vi "FiletxtOpen.vi"(6 "Tips":refnum<vi>, 7 "Language":u32, 8 "ProgressBar":refnum<vi>, 9 "ProgressNum":refnum<vi>, 10 "MessageLinCnt":refnum<vi>, 11 "file path (dialog if empty)":path caption="文件路径 （空时为对话框）") -> (0 "PathOut":path, 1 "重构的Data数组":u32[][](array[numeric]), 2 "统计数量":string[](array[string]), 3 "报文ID":string[](array[string]), 4 "BaseTimeCluster":T1, 5 "CAN报文统计":string[][](array[string]))   [LabVIEW 2015]
uses:
  <vilib>/Utility/file.llb/Read Delimited Spreadsheet (string).vi
  <vilib>/regexp/Match Regular Expression.xnode
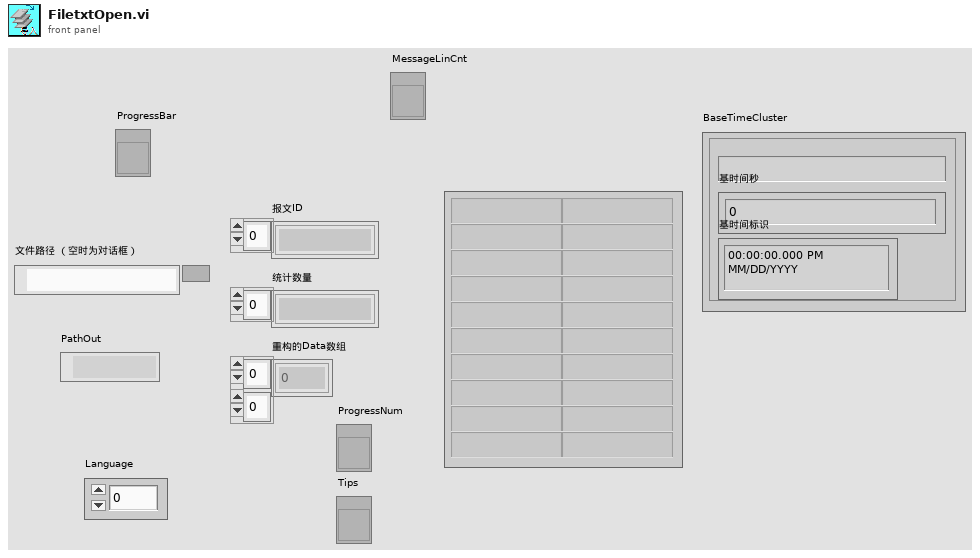
[diagram p1: front panel]
types:
  T1 = cluster{"基时间字符串":string, "基时间秒":dbl, "基时间标识":timestamp}
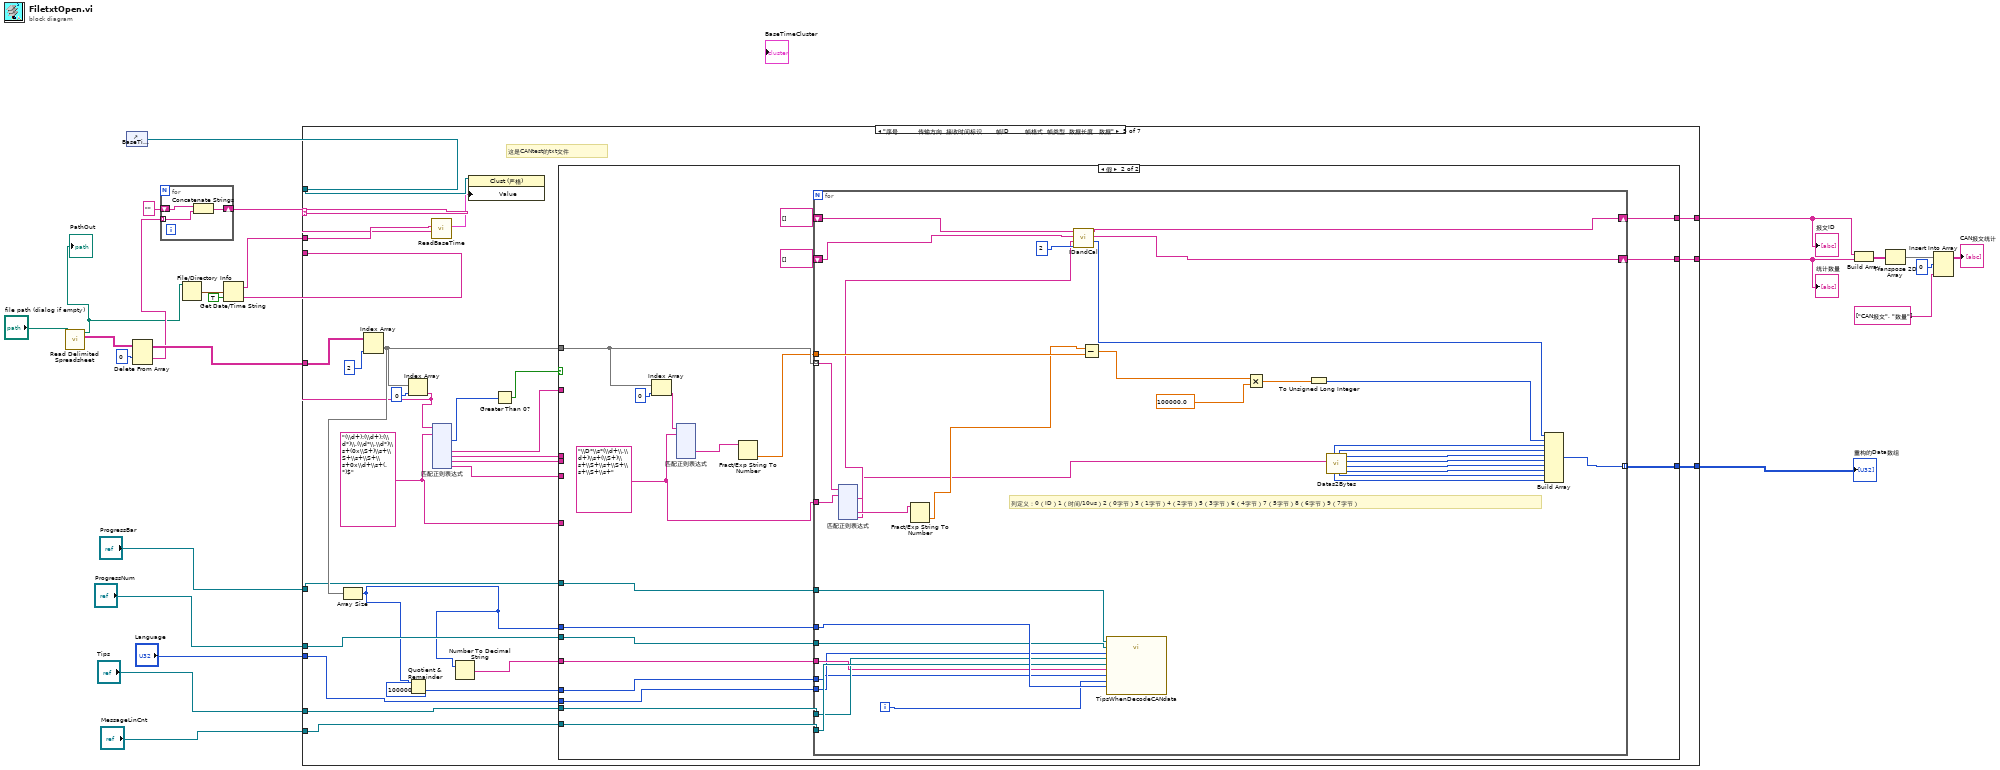
[diagram p0: block diagram]
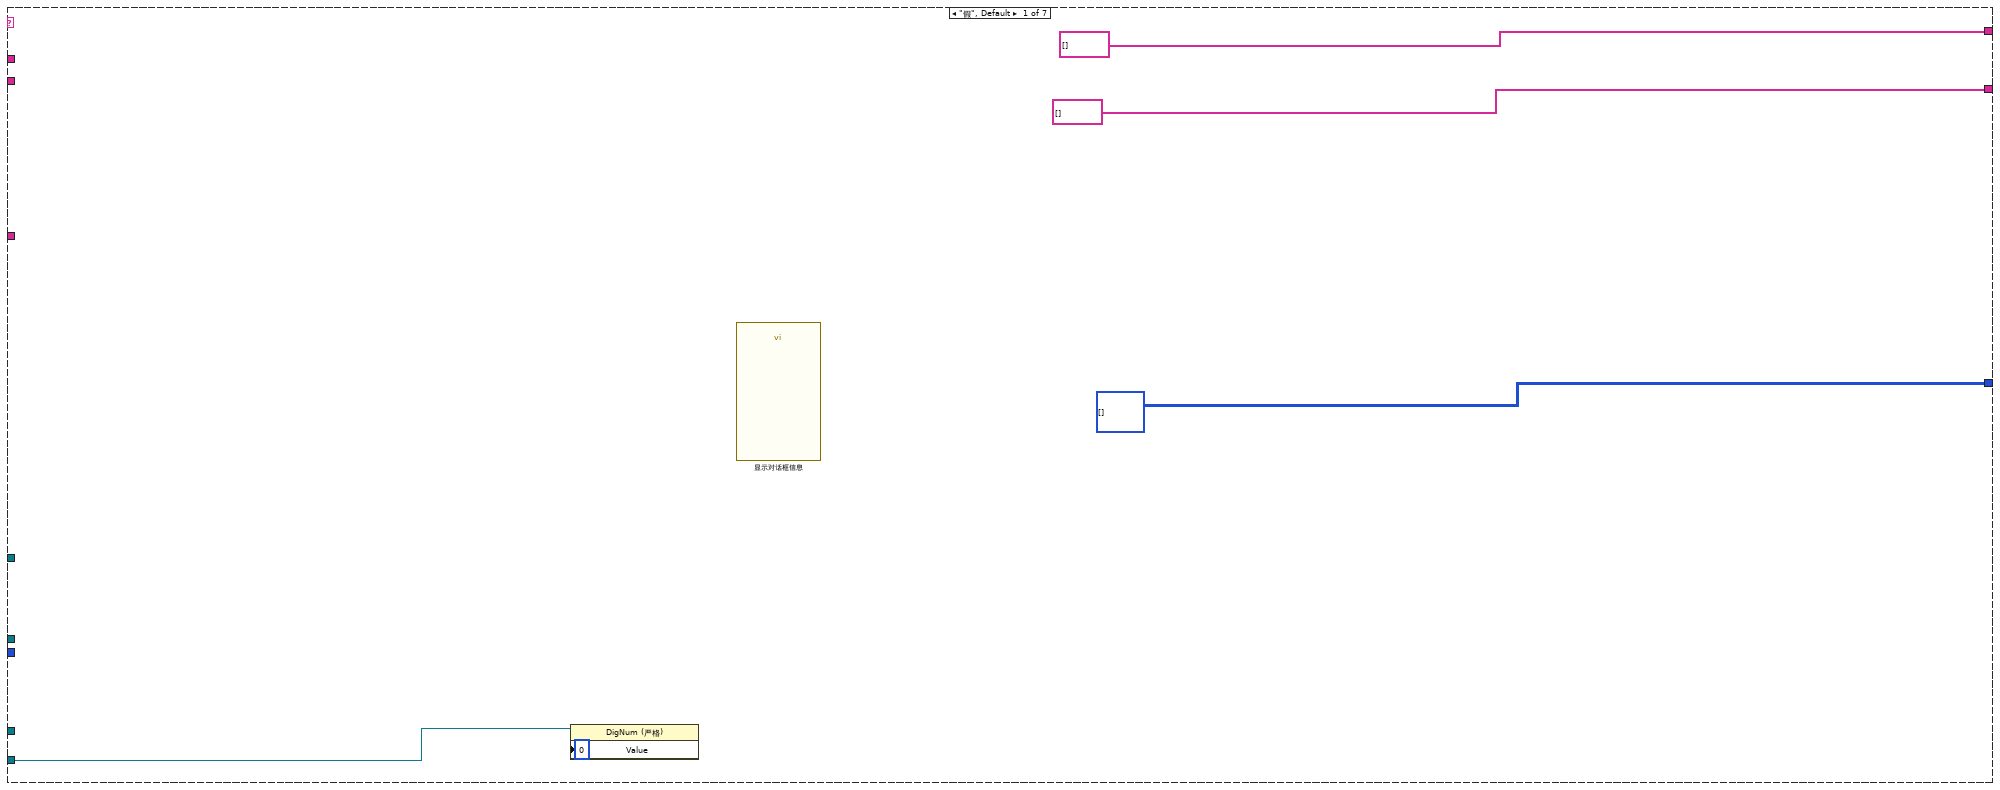
[diagram p2: hidden frame]
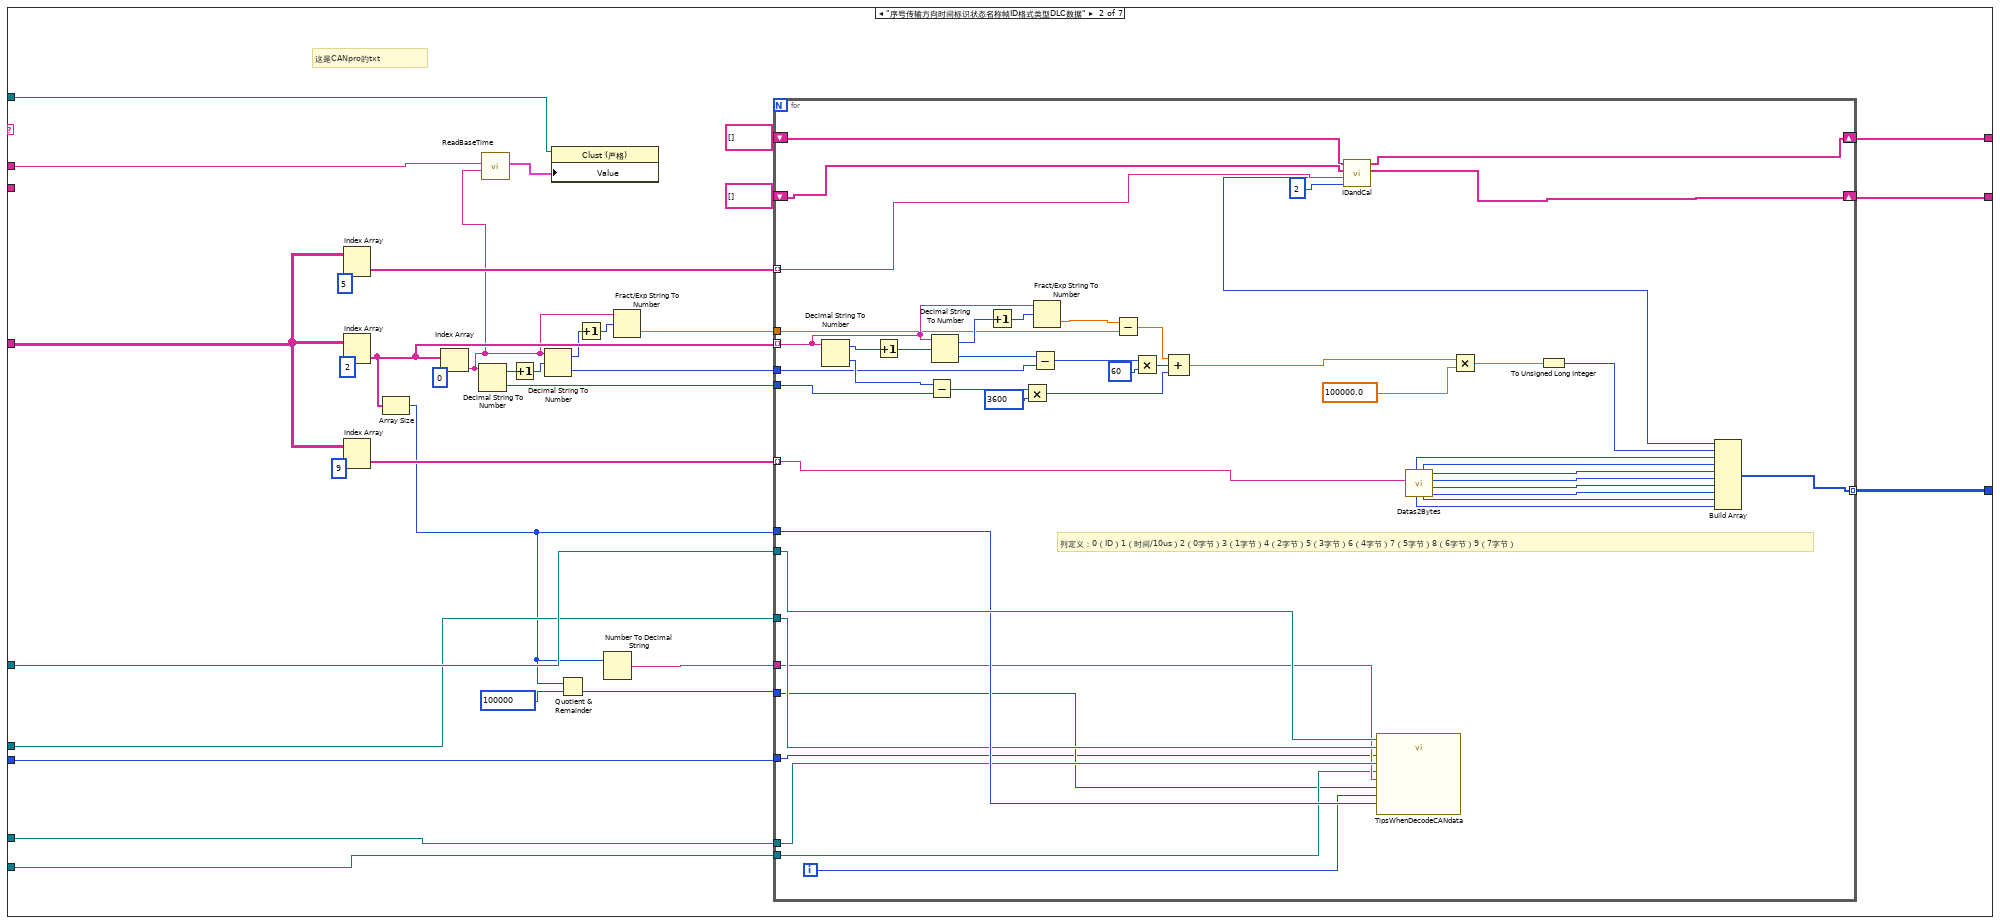
[diagram p3: hidden frame]
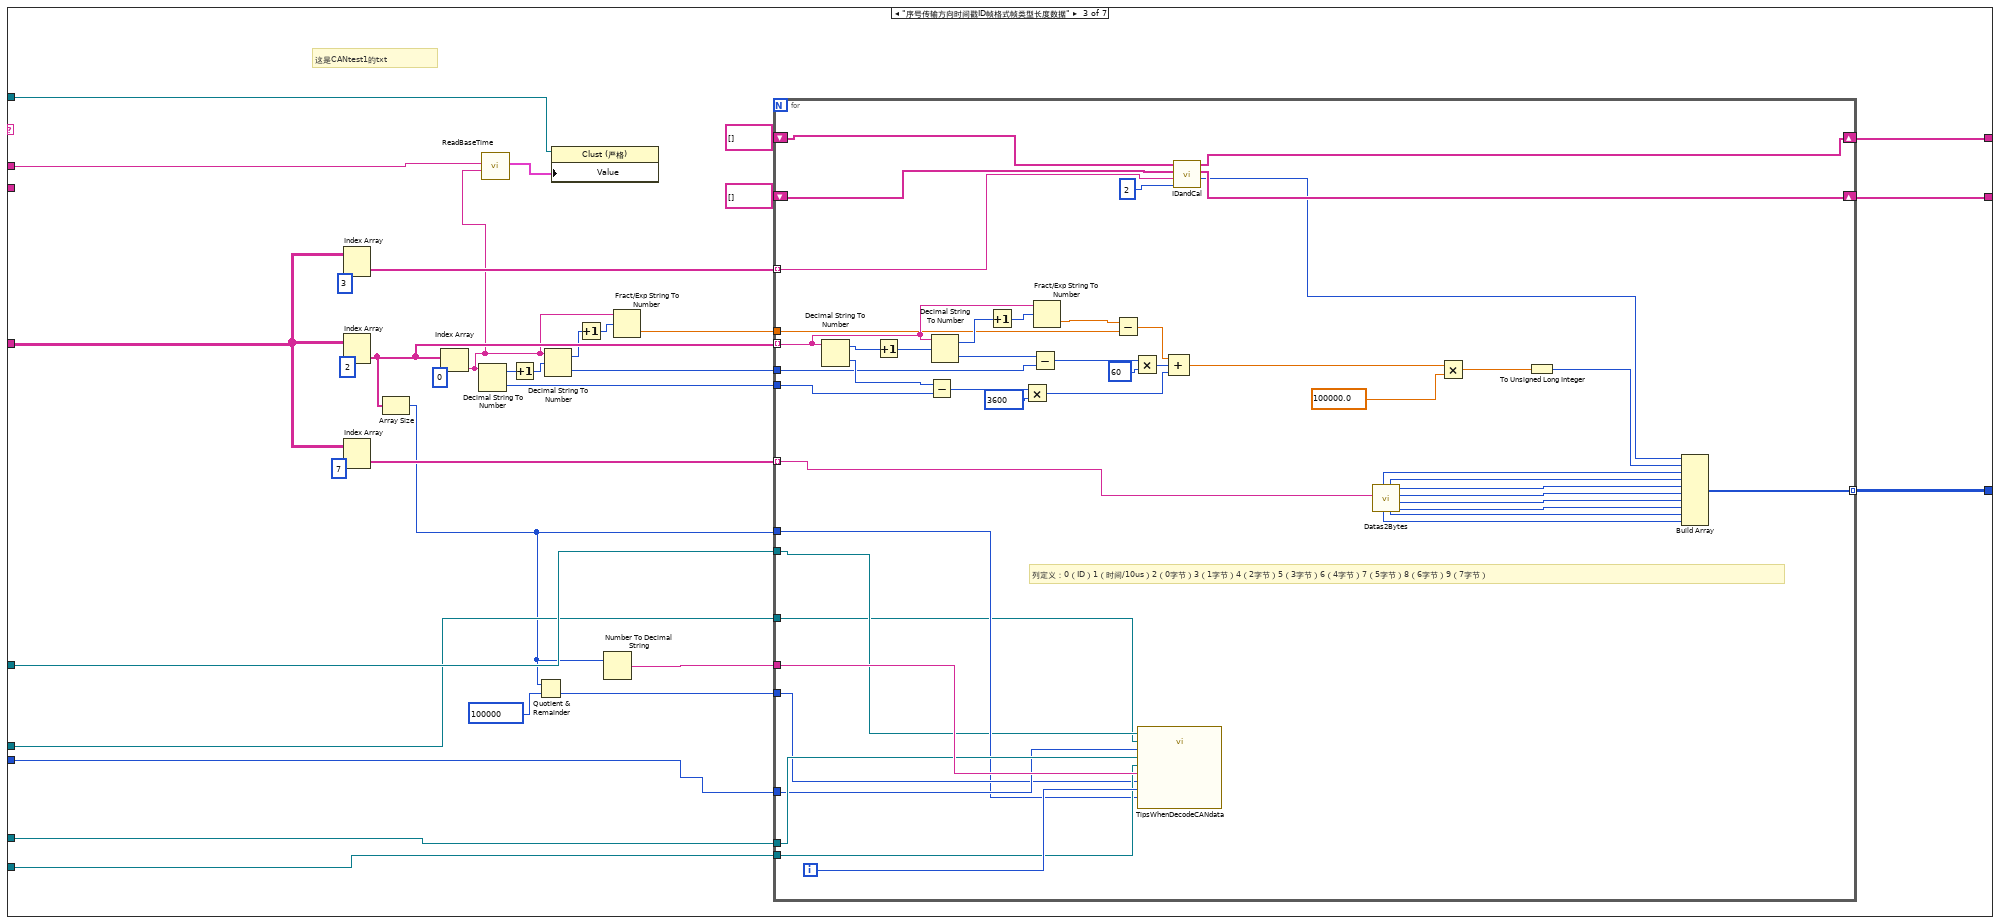
[diagram p4: hidden frame]
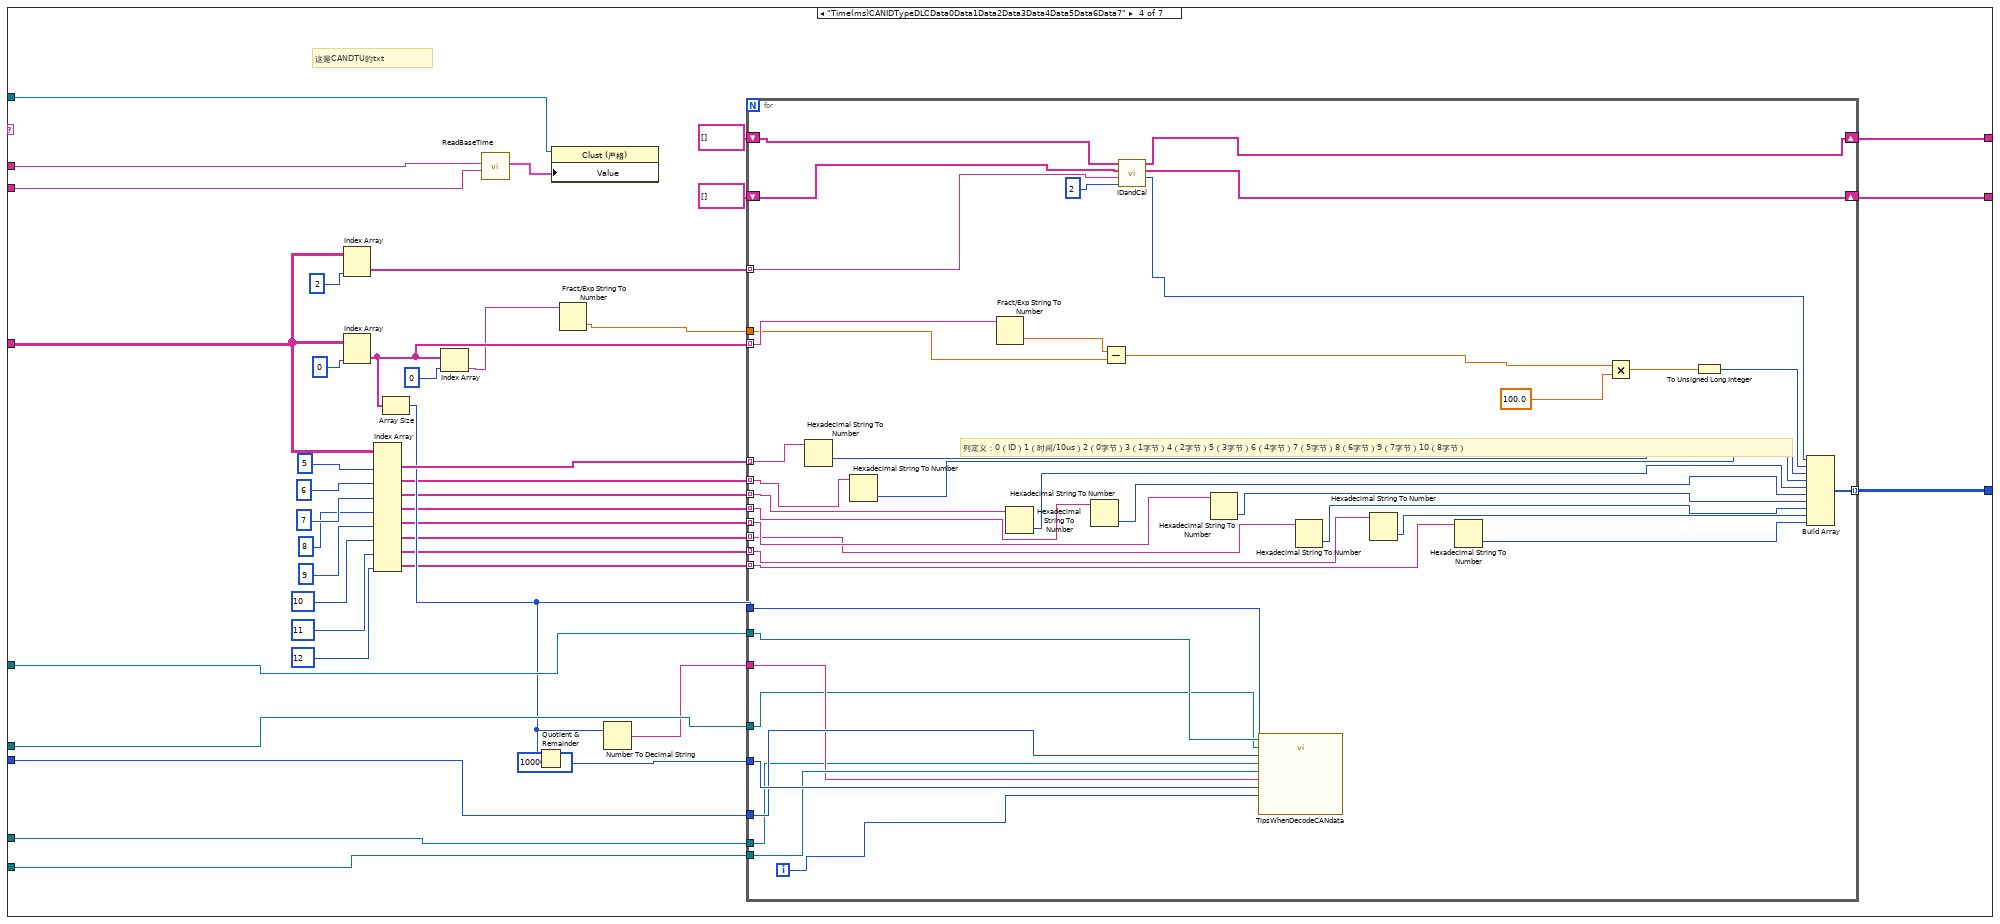
[diagram p5: hidden frame]
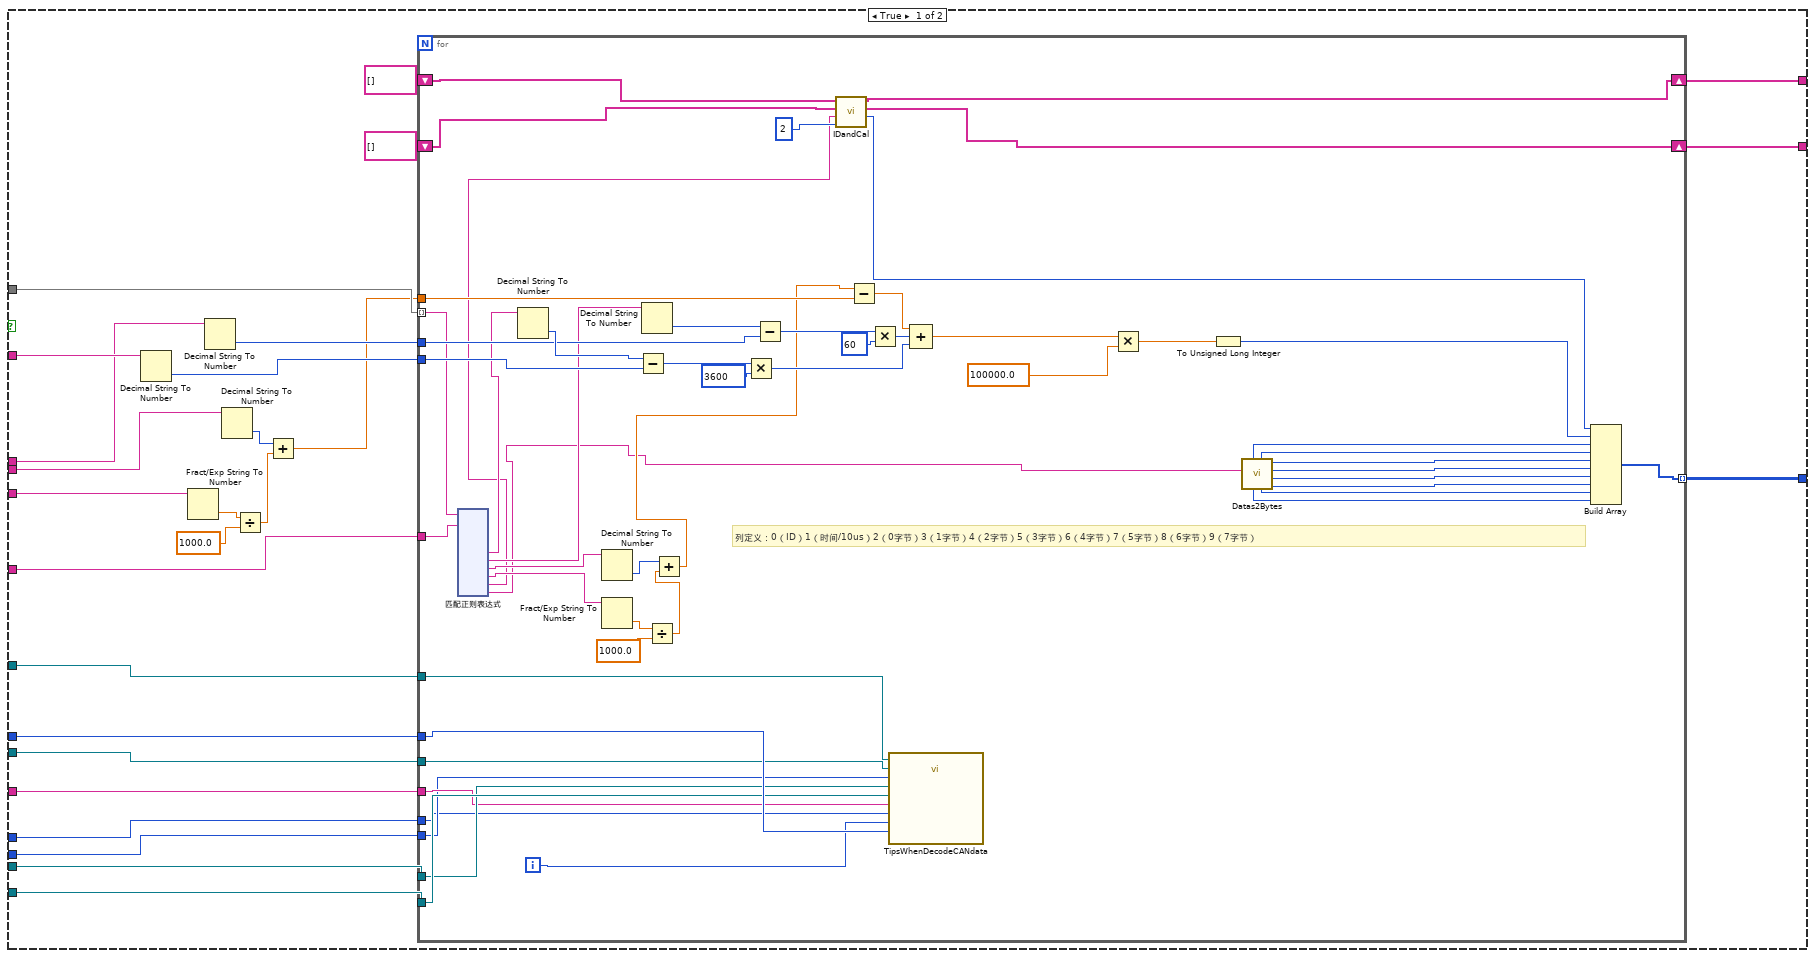
[diagram p6: hidden frame]
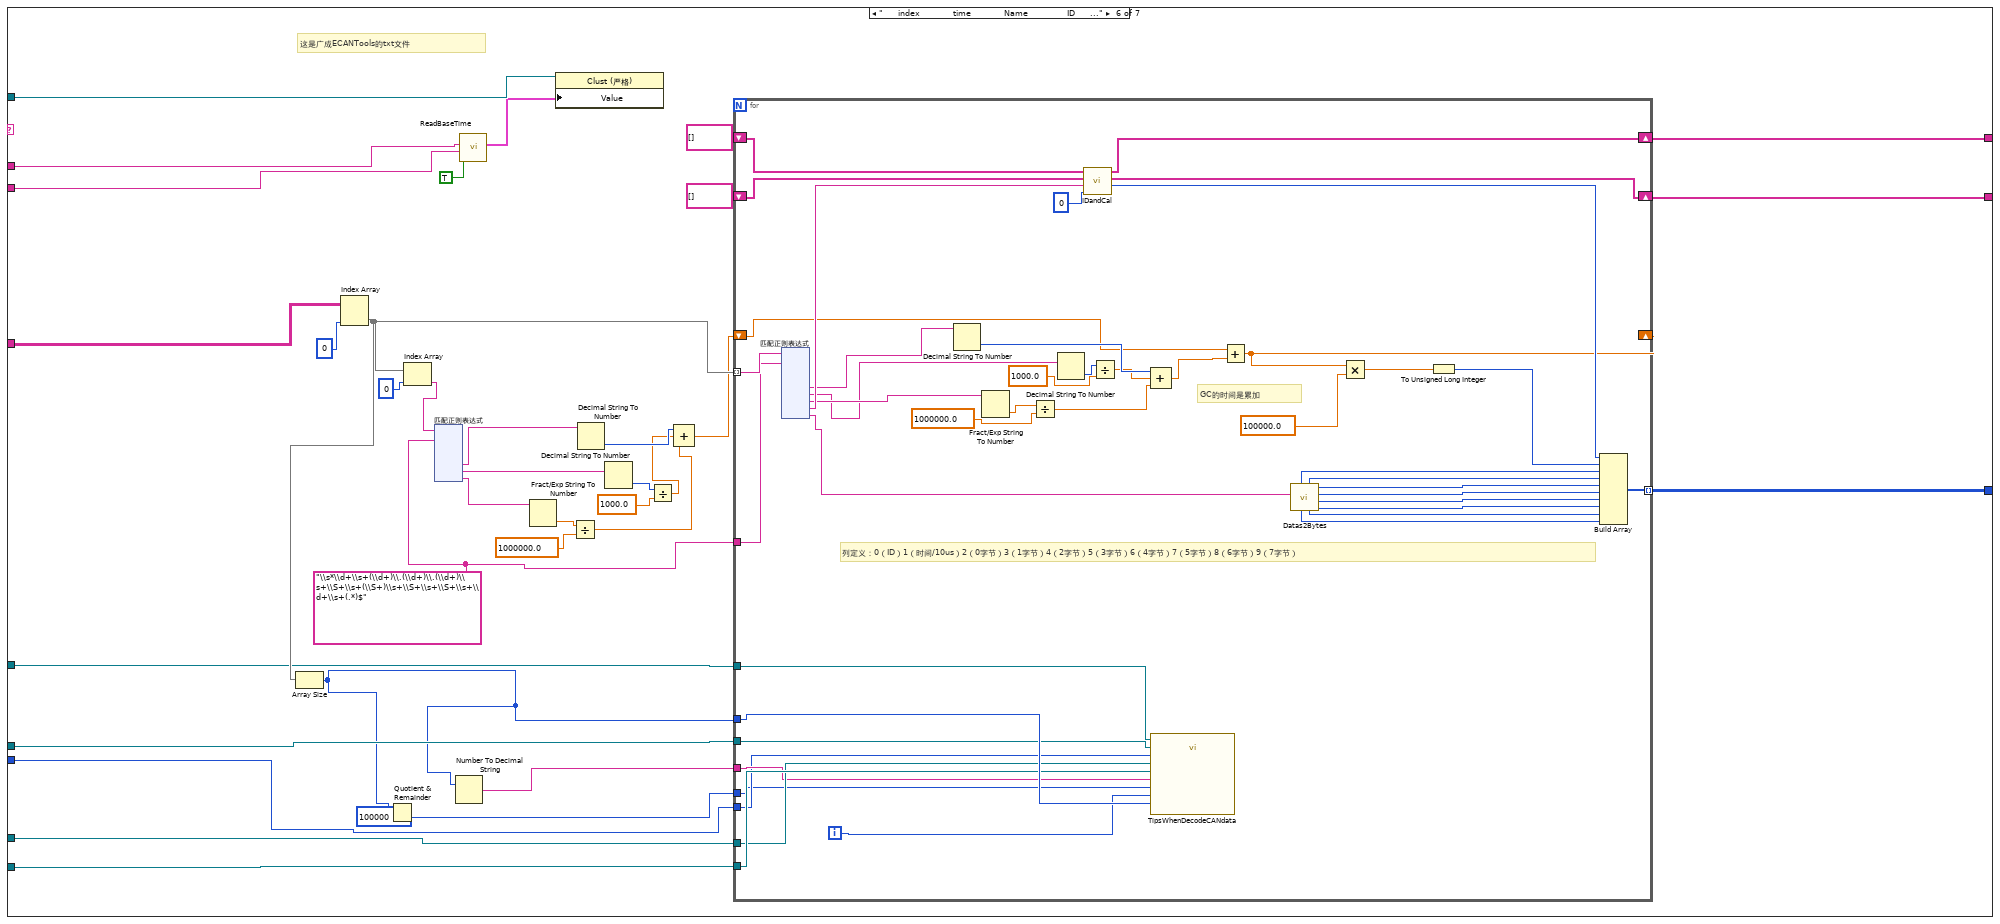
[diagram p7: hidden frame]
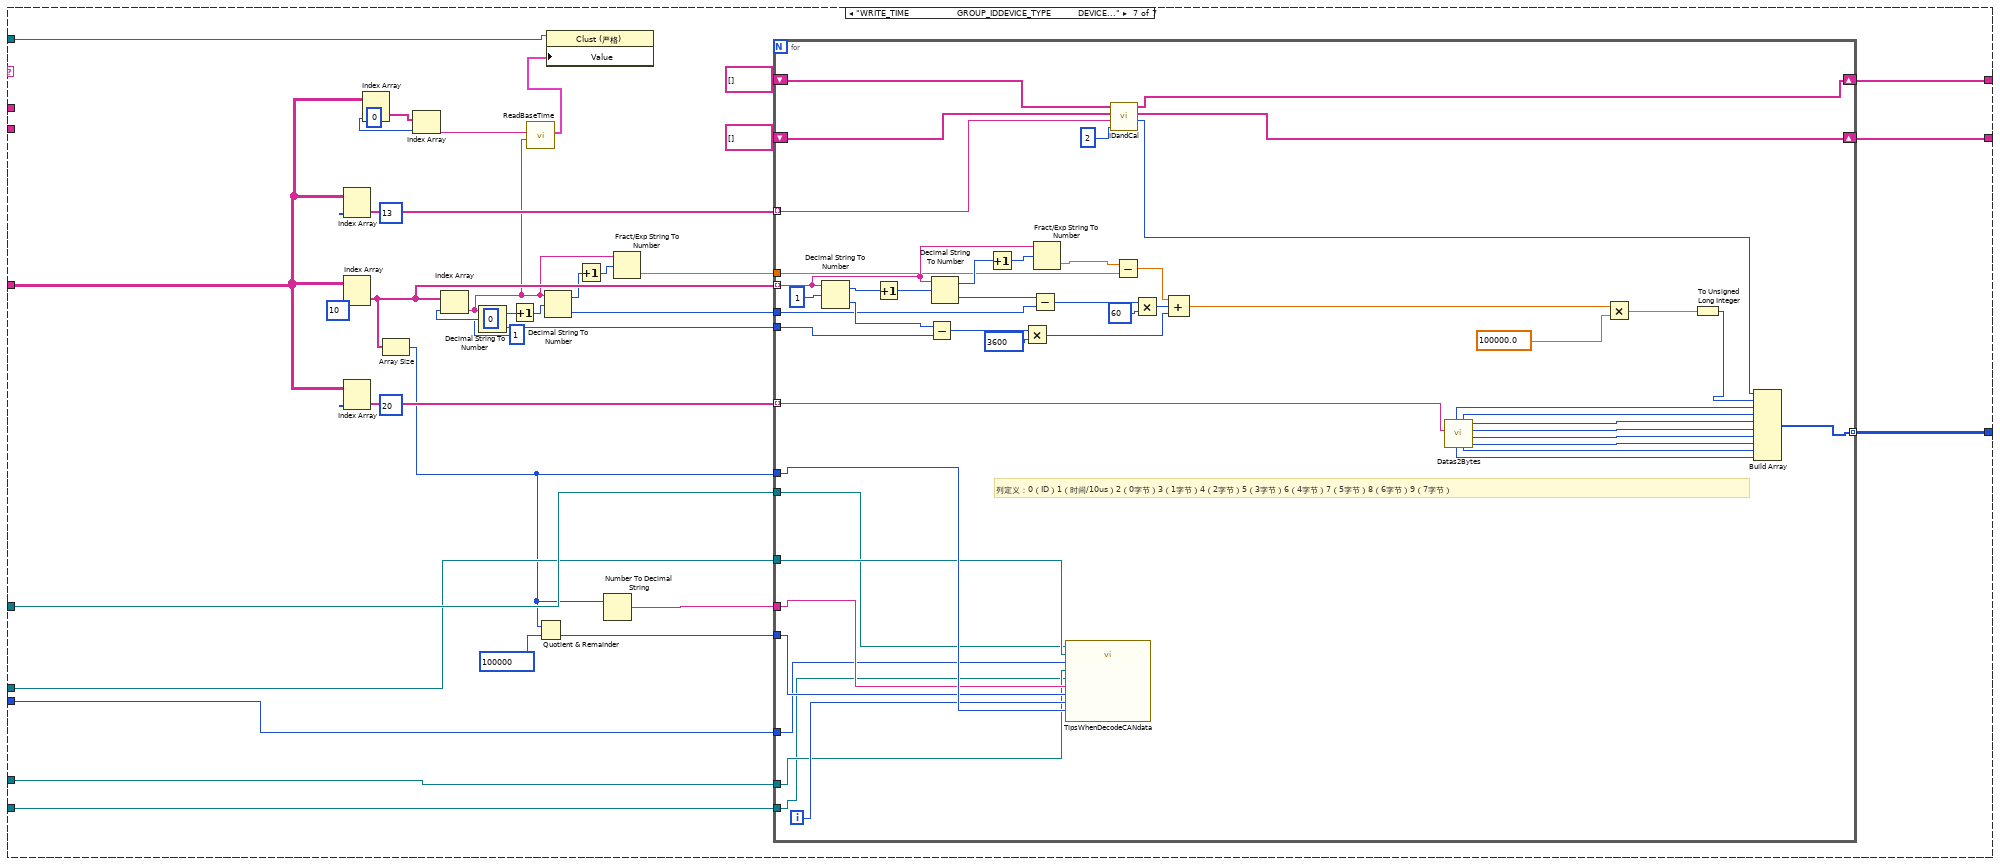
[diagram p8: hidden frame]
diagram:
  n1 = call-poly <vilib>:"Read Delimited Spreadsheet.vi"("file path (dialog if empty)"="file path (dialog if empty)") -> ("new file path (Not A Path if cancelled)"=w6:path, "all rows"=w16:string[][])  [unwired: 9 in, 4 out]
  "PathOut" <- w6
  n2 = control-ref of="BaseTimeCluster"() -> (w4:refnum<vi>)
  n3 = Delete From Array(array=w16, index (row)=0 ("索引 (行)")) -> (deleted portion=w9:string[], array with subset deleted=w25:string[][])  [unwired: 2 in]
  n4 = for {
    tunnel: w9 -> [w28] mode=indexing
    shift-right: [w29] -> w8
    shift-left: "" -> [w27]
    n5 = Concatenate Strings(w27, w28) -> (w29:string)
  }
  n6 = File/Directory Info(path=w6) -> (last mod=w7:timestamp)  [unwired: 1 in, 6 out]
  n7 = Get Date/Time String(seconds (now)=w7, want seconds? (F)=TRUE ("需要秒？(F)")) -> (date string=w5:string, time string=w3:string)  [unwired: 1 in]
  n8 = case shown="\"序号          传输方向  接收时间标识       帧ID        帧格式  帧类型  数据长度   数据\"" w8 {
    tunnel: [u32[][] [] w67 w148 w238 w305 w948 w1266] -> w26
    tunnel: w25 -> [_ w65 w146 w236 w304 w947 w1237]
    tunnel: [string[] [] w49 w130 w227 w300 w941 w1249] -> w19
    tunnel: [string[] [] w48 w129 w226 w299 w940 w1248] -> w18
    tunnel: "ProgressBar" -> [_ w47 w128 w225 w298 w939 w1247]
    tunnel: "ProgressNum" -> [_ w46 w127 w224 w297 w938 w1246]
    tunnel: "Tips" -> [_ w43 w124 w221 w294 w935 w1243]
    tunnel: "MessageLinCnt" -> [w31 w36 w117 w215 w282 w926 w1232]
    tunnel: w5 -> [_ w38 w119 w217 w286 w930 _]
    tunnel: w4 -> [_ w37 w118 w216 w284 w928 w1234]
    tunnel: w3 -> [_ _ _ w199 _ w914 _]
    tunnel: "Language" -> [_ w35 w116 w197 w281 w925 w1231]
    frame "假", Default {
      n9 = property class="DigNum (严格)"(reference=w31, "Value"=0 ("值")) -> ()  [unwired: 1 in, 2 out]
      n10 = call "显示对话框信息"() -> ()  [unwired: 10 in, 2 out]
    }
    frame "序号传输方向时间标识状态名称帧ID格式类型DLC数据" {
      # "这是CANpro的txt"
      n11 = Index Array(array=w65, index (col)=5 ("禁用的索引 (列)")) -> (element=w66:string[])  [unwired: 1 in]
      n12 = Index Array(array=w65, index (col)=2 ("禁用的索引 (列)")) -> (element=w56:string[])  [unwired: 1 in]
      n13 = Index Array(array=w65, index (col)=9 ("禁用的索引 (列)")) -> (element=w61:string[])  [unwired: 1 in]
      n14 = Array Size(array=w56) -> (size(s)=w41:i32)
      n15 = Index Array(array=w56, index=0 ("索引")) -> (element=w40:string)
      n16 = Decimal String To Number(string=w40) -> (offset past number=w53:i32, number=w57:i32)  [unwired: 2 in]
      n17 = call "ReadBaseTime.vi"("时间字符"=w40, "日期字符"=w38) -> ("基时间簇"=w39:T1)  [unwired: 7 in]
      n18 = Increment(x=w53) -> (x+1=w54:i32)
      n19 = Decimal String To Number(string=w40, offset=w54) -> (offset past number=w55:i32, number=w58:i32)  [unwired: 1 in]
      n20 = property class="Clust (严格)"(reference=w37, "Value"=w39) -> ()  [unwired: 1 in, 2 out]
      n21 = Quotient & Remainder(x=w41, y=100000) -> (floor(x/y)=w44:i32)  [unwired: 1 out]
      n22 = Increment(x=w55) -> (x+1=w59:i32)
      n23 = Number To Decimal String(number=w41) -> (decimal integer string=w42:string)  [unwired: 1 in]
      n24 = Fract/Exp String To Number(string=w40, offset=w59) -> (number=w60:dbl)  [unwired: 2 in, 1 out]
      n25 = for {
        tunnel: w56 -> [w101] mode=indexing
        tunnel: w57 -> [w111]
        tunnel: w58 -> [w107]
        tunnel: w60 -> [w99]
        tunnel: w61 -> [w68] mode=indexing
        tunnel: [w71] -> w67 mode=indexing
        shift-right: [w84] -> w49
        shift-left: string[] [] -> [w80]
        shift-right: [w85] -> w48
        shift-left: string[] [] -> [w81]
        tunnel: w66 -> [w82] mode=indexing
        tunnel: w41 -> [w93]
        tunnel: w47 -> [w94]
        tunnel: w46 -> [w92]
        tunnel: w44 -> [w87]
        tunnel: w43 -> [w91]
        tunnel: w42 -> [w90]
        tunnel: w36 -> [w89]
        tunnel: w35 -> [w86]
        i -> [w88]
        # "列定义：0（ID）1（时间/10us）2（0字节）3（1字节）4（2字节）5（3字节）6（4字节）7（5字节）8（6字节）9（7字节）"
        n26 = Decimal String To Number(string=w101) -> (offset past number=w113:i32, number=w112:i32)  [unwired: 2 in]
        n27 = Increment(x=w113) -> (x+1=w114:i32)
        n28 = Subtract(x=w112, y=w111) -> (x-y=w110:i32)
        n29 = Decimal String To Number(string=w101, offset=w114) -> (offset past number=w115:i32, number=w108:i32)  [unwired: 1 in]
        n30 = Increment(x=w115) -> (x+1=w102:i32)
        n31 = Multiply(x=w110, y=3600) -> (x*y=w103:i32)
        n32 = Subtract(x=w108, y=w107) -> (x-y=w106:i32)
        n33 = Fract/Exp String To Number(string=w101, offset=w102) -> (number=w100:dbl)  [unwired: 2 in, 1 out]
        n34 = Subtract(x=w100, y=w99) -> (x-y=w98:dbl)
        n35 = Multiply(x=w106, y=60) -> (x*y=w104:i32)
        n36 = Compound Arithmetic op=ADD(w98, w104, w103) -> (w97:dbl)
        n37 = call "IDandCal.vi"("ID列表In"=w80, "数量统计in"=w81, "ID输入"=w82, "偏移量(0)"=2) -> ("ID列表"=w84:string[], "数量统计"=w85:string[], "ID输出"=w70:u32)  [unwired: 3 in]
        n38 = call "TipsWhenDecodeCANdata.vi"("ProgressBar"=w94, "AllRowsNum"=w93, "i"=w88, "ProgressNum"=w92, "Language"=w86, "Tips"=w91, "MessageLinCnt"=w89, "txtAllRowsNum"=w90, "RowsLevel"=w87) -> ()  [unwired: 7 in]
        n39 = call "Datas2Bytes.vi"("DATAs"=w68) -> ("Data5"=w74:u32, "Data4"=w75:u32, "Data3"=w76:u32, "Data2"=w77:u32, "Data6"=w73:u32, "Data1"=w78:u32, "Data7"=w72:u32, "Data0"=w79:u32)  [unwired: 3 in]
        n40 = Multiply(x=w97, y=100000.0) -> (x*y=w95:dbl)
        n41 = To Unsigned Long Integer(number=w95) -> (unsigned 32bit integer=w69:u32)
        n42 = Build Array(w70, w69, w79, w78, w77, w76, w75, w74, w73, w72) -> (w71:u32[])
      }
    }
    frame "序号传输方向时间戳ID帧格式帧类型长度数据" {
      # "这是CANtest1的txt"
      n43 = Index Array(array=w146, index (col)=3 ("禁用的索引 (列)")) -> (element=w147:string[])  [unwired: 1 in]
      n44 = Index Array(array=w146, index (col)=2 ("禁用的索引 (列)")) -> (element=w137:string[])  [unwired: 1 in]
      n45 = Index Array(array=w146, index (col)=7 ("禁用的索引 (列)")) -> (element=w142:string[])  [unwired: 1 in]
      n46 = Array Size(array=w137) -> (size(s)=w122:i32)
      n47 = Index Array(array=w137, index=0 ("索引")) -> (element=w121:string)
      n48 = Decimal String To Number(string=w121) -> (offset past number=w134:i32, number=w138:i32)  [unwired: 2 in]
      n49 = call "ReadBaseTime.vi"("时间字符"=w121, "日期字符"=w119) -> ("基时间簇"=w120:T1)  [unwired: 7 in]
      n50 = Increment(x=w134) -> (x+1=w135:i32)
      n51 = Quotient & Remainder(x=w122, y=100000) -> (floor(x/y)=w125:i32)  [unwired: 1 out]
      n52 = Decimal String To Number(string=w121, offset=w135) -> (offset past number=w136:i32, number=w139:i32)  [unwired: 1 in]
      n53 = property class="Clust (严格)"(reference=w118, "Value"=w120) -> ()  [unwired: 1 in, 2 out]
      n54 = Increment(x=w136) -> (x+1=w140:i32)
      n55 = Number To Decimal String(number=w122) -> (decimal integer string=w123:string)  [unwired: 1 in]
      n56 = Fract/Exp String To Number(string=w121, offset=w140) -> (number=w141:dbl)  [unwired: 2 in, 1 out]
      n57 = for {
        tunnel: w137 -> [w182] mode=indexing
        tunnel: w138 -> [w192]
        tunnel: w139 -> [w188]
        tunnel: w141 -> [w180]
        tunnel: w142 -> [w149] mode=indexing
        tunnel: [w152] -> w148 mode=indexing
        shift-right: [w164] -> w130
        shift-left: string[] [] -> [w162]
        shift-right: [w163] -> w129
        shift-left: string[] [] -> [w161]
        tunnel: w147 -> [w165] mode=indexing
        tunnel: w122 -> [w169]
        tunnel: w128 -> [w168]
        tunnel: w127 -> [w167]
        tunnel: w125 -> [w170]
        tunnel: w124 -> [w172]
        tunnel: w123 -> [w175]
        tunnel: w117 -> [w173]
        tunnel: w116 -> [w171]
        i -> [w174]
        # "列定义：0（ID）1（时间/10us）2（0字节）3（1字节）4（2字节）5（3字节）6（4字节）7（5字节）8（6字节）9（7字节）"
        n58 = Decimal String To Number(string=w182) -> (offset past number=w194:i32, number=w193:i32)  [unwired: 2 in]
        n59 = Increment(x=w194) -> (x+1=w195:i32)
        n60 = Subtract(x=w193, y=w192) -> (x-y=w191:i32)
        n61 = Decimal String To Number(string=w182, offset=w195) -> (offset past number=w196:i32, number=w189:i32)  [unwired: 1 in]
        n62 = Increment(x=w196) -> (x+1=w183:i32)
        n63 = Multiply(x=w191, y=3600) -> (x*y=w184:i32)
        n64 = Subtract(x=w189, y=w188) -> (x-y=w187:i32)
        n65 = Fract/Exp String To Number(string=w182, offset=w183) -> (number=w181:dbl)  [unwired: 2 in, 1 out]
        n66 = Subtract(x=w181, y=w180) -> (x-y=w179:dbl)
        n67 = Multiply(x=w187, y=60) -> (x*y=w185:i32)
        n68 = call "TipsWhenDecodeCANdata.vi"("ProgressBar"=w168, "AllRowsNum"=w169, "i"=w174, "ProgressNum"=w167, "Language"=w171, "Tips"=w172, "MessageLinCnt"=w173, "txtAllRowsNum"=w175, "RowsLevel"=w170) -> ()  [unwired: 7 in]
        n69 = Compound Arithmetic op=ADD(w179, w185, w184) -> (w178:dbl)
        n70 = call "IDandCal.vi"("ID列表In"=w162, "数量统计in"=w161, "ID输入"=w165, "偏移量(0)"=2) -> ("ID列表"=w164:string[], "数量统计"=w163:string[], "ID输出"=w151:u32)  [unwired: 3 in]
        n71 = call "Datas2Bytes.vi"("DATAs"=w149) -> ("Data5"=w155:u32, "Data4"=w156:u32, "Data3"=w157:u32, "Data2"=w158:u32, "Data6"=w154:u32, "Data1"=w159:u32, "Data7"=w153:u32, "Data0"=w160:u32)  [unwired: 3 in]
        n72 = Multiply(x=w178, y=100000.0) -> (x*y=w176:dbl)
        n73 = To Unsigned Long Integer(number=w176) -> (unsigned 32bit integer=w150:u32)
        n74 = Build Array(w151, w150, w160, w159, w158, w157, w156, w155, w154, w153) -> (w152:u32[])
      }
    }
    frame "Time(ms)CANIDTypeDLCData0Data1Data2Data3Data4Data5Data6Data7" {
      # "这是CANDTU的txt"
      n75 = Index Array(array=w236, index (col)=2 ("禁用的索引 (列)")) -> (element=w237:string[])  [unwired: 1 in]
      n76 = Index Array(array=w236, index (col)=0 ("禁用的索引 (列)")) -> (element=w231:string[])  [unwired: 1 in]
      n77 = Index Array(array=w236, index (col) #1=5 ("禁用的索引 (列)"), index (col) #2=6 ("禁用的索引 (列)"), index (col) #3=7 ("禁用的索引 (列)"), index (col) #4=8 ("禁用的索引 (列)"), index (col) #5=9 ("禁用的索引 (列)"), index (col) #6=10 ("禁用的索引 (列)"), index (col) #7=11 ("禁用的索引 (列)"), index (col) #8=12 ("禁用的索引 (列)")) -> (element #1=w232:string[], element #2=w207:string[], element #3=w206:string[], element #4=w205:string[], element #5=w204:string[], element #6=w203:string[], element #7=w202:string[], element #8=w201:string[])  [unwired: 8 in]
      n78 = Array Size(array=w231) -> (size(s)=w219:i32)
      n79 = Index Array(array=w231, index=0 ("索引")) -> (element=w198:string)
      n80 = call "ReadBaseTime.vi"("时间字符"=w199, "日期字符"=w217) -> ("基时间簇"=w218:T1)  [unwired: 7 in]
      n81 = Quotient & Remainder(x=w219, y=100000) -> (floor(x/y)=w222:i32)  [unwired: 1 out]
      n82 = property class="Clust (严格)"(reference=w216, "Value"=w218) -> ()  [unwired: 1 in, 2 out]
      n83 = Fract/Exp String To Number(string=w198) -> (number=w200:dbl)  [unwired: 3 in, 1 out]
      n84 = Number To Decimal String(number=w219) -> (decimal integer string=w220:string)  [unwired: 1 in]
      n85 = for {
        tunnel: w231 -> [w278] mode=indexing
        tunnel: w200 -> [w276]
        tunnel: w232 -> [w263] mode=indexing
        tunnel: [w267] -> w238 mode=indexing
        shift-right: [w243] -> w227
        shift-left: string[] [] -> [w242]
        shift-right: [w244] -> w226
        shift-left: string[] [] -> [w240]
        tunnel: w237 -> [w241] mode=indexing
        tunnel: w219 -> [w254]
        tunnel: w225 -> [w247]
        tunnel: w224 -> [w246]
        tunnel: w222 -> [w252]
        tunnel: w221 -> [w248]
        tunnel: w220 -> [w249]
        tunnel: w215 -> [w250]
        tunnel: w207 -> [w262] mode=indexing
        tunnel: w206 -> [w261] mode=indexing
        tunnel: w205 -> [w260] mode=indexing
        tunnel: w204 -> [w259] mode=indexing
        tunnel: w203 -> [w258] mode=indexing
        tunnel: w202 -> [w257] mode=indexing
        tunnel: w201 -> [w256] mode=indexing
        tunnel: w197 -> [w251]
        i -> [w253]
        # "列定义：0（ID）1（时间/10us）2（0字节）3（1字节）4（2字节）5（3字节）6（4字节）7（5字节）8（6字节）9（7字节）10（8字节）"
        n86 = Hexadecimal String To Number(string=w263) -> (number=w275:u32)  [unwired: 2 in, 1 out]
        n87 = Hexadecimal String To Number(string=w262) -> (number=w274:u32)  [unwired: 2 in, 1 out]
        n88 = Fract/Exp String To Number(string=w278) -> (number=w277:dbl)  [unwired: 3 in, 1 out]
        n89 = Hexadecimal String To Number(string=w261) -> (number=w273:u32)  [unwired: 2 in, 1 out]
        n90 = Hexadecimal String To Number(string=w260) -> (number=w272:u32)  [unwired: 2 in, 1 out]
        n91 = Subtract(x=w277, y=w276) -> (x-y=w255:dbl)
        n92 = call "IDandCal.vi"("ID列表In"=w242, "数量统计in"=w240, "ID输入"=w241, "偏移量(0)"=2) -> ("ID列表"=w243:string[], "数量统计"=w244:string[], "ID输出"=w239:u32)  [unwired: 3 in]
        n93 = Hexadecimal String To Number(string=w259) -> (number=w271:u32)  [unwired: 2 in, 1 out]
        n94 = call "TipsWhenDecodeCANdata.vi"("ProgressBar"=w247, "AllRowsNum"=w254, "i"=w253, "ProgressNum"=w246, "Language"=w251, "Tips"=w248, "MessageLinCnt"=w250, "txtAllRowsNum"=w249, "RowsLevel"=w252) -> ()  [unwired: 7 in]
        n95 = Hexadecimal String To Number(string=w258) -> (number=w270:u32)  [unwired: 2 in, 1 out]
        n96 = Hexadecimal String To Number(string=w257) -> (number=w269:u32)  [unwired: 2 in, 1 out]
        n97 = Hexadecimal String To Number(string=w256) -> (number=w268:u32)  [unwired: 2 in, 1 out]
        n98 = Multiply(x=w255, y=100.0) -> (x*y=w265:dbl)
        n99 = To Unsigned Long Integer(number=w265) -> (unsigned 32bit integer=w264:u32)
        n100 = Build Array(w239, w264, w275, w274, w273, w272, w271, w270, w269, w268) -> (w267:u32[])
      }
    }
    frame "序号          传输方向  接收时间标识       帧ID        帧格式  帧类型  数据长度   数据" {
      w287 = "(\\d+):(\\d+):(\\d*)\\.(\\d*\\.\\d*)\\s+(0x\\S+)\\s+\\S+\\s+\\S+\\s+0x\\d+\\s+(.*)$"
      # "这是CANtest的txt文件"
      n101 = Index Array(array=w304, index (col)=2 ("禁用的索引 (列)")) -> (element=w303:string[])  [unwired: 1 in]
      n102 = Array Size(array=w303) -> (size(s)=w292:i32)
      n103 = Index Array(array=w303, index=0 ("索引")) -> (element=w285:string)
      n104 = Quotient & Remainder(x=w292, y=100000) -> (floor(x/y)=w295:i32)  [unwired: 1 out]
      n105 = call "ReadBaseTime.vi"("时间字符"=w285, "日期字符"=w286) -> ("基时间簇"=w283:T1)  [unwired: 7 in]
      n106 = xnode "匹配正则表达式"("输入字符串"=w285, "正则表达式"=w287) -> ("匹配后偏移量"=w280:i32, "子匹配 1"=w291:string, "子匹配 2"=w290:string, "子匹配 3"=w289:string, "子匹配 4"=w288:string)  [unwired: 4 in, 4 out]
      n107 = Number To Decimal String(number=w292) -> (decimal integer string=w293:string)  [unwired: 1 in]
      n108 = property class="Clust (严格)"(reference=w284, "Value"=w283) -> ()  [unwired: 1 in, 2 out]
      n109 = Greater Than 0?(x=w280) -> (x > 0?=w279:bool)
      n110 = case shown="假" w279 {
        tunnel: [w331 w524] -> w305
        tunnel: w303 -> [w326 w509]
        tunnel: [w325 w521] -> w300
        tunnel: [w324 w520] -> w299
        tunnel: w298 -> [w323 w519]
        tunnel: w297 -> [w322 w518]
        tunnel: w295 -> [w321 w517]
        tunnel: w294 -> [w320 w516]
        tunnel: w293 -> [w319 w515]
        tunnel: w292 -> [w318 w514]
        tunnel: w291 -> [w317 _]
        tunnel: w290 -> [w316 _]
        tunnel: w289 -> [w315 _]
        tunnel: w288 -> [w314 _]
        tunnel: w287 -> [w308 _]
        tunnel: w282 -> [w307 w513]
        tunnel: w281 -> [w306 w512]
        frame True {
          n111 = Decimal String To Number(string=w317) -> (number=w327:i32)  [unwired: 2 in, 1 out]
          n112 = Fract/Exp String To Number(string=w314) -> (number=w312:dbl)  [unwired: 3 in, 1 out]
          n113 = Decimal String To Number(string=w316) -> (number=w328:i32)  [unwired: 2 in, 1 out]
          n114 = Decimal String To Number(string=w315) -> (number=w309:i32)  [unwired: 2 in, 1 out]
          n115 = Divide(x=w312, y=1000.0) -> (x/y=w310:dbl)
          n116 = Add(x=w309, y=w310) -> (x+y=w313:dbl)
          n117 = for {
            tunnel: w326 -> [w369] mode=indexing
            tunnel: w327 -> [w383]
            tunnel: w328 -> [w379]
            tunnel: w313 -> [w374]
            tunnel: [w335] -> w331 mode=indexing
            shift-right: [w347] -> w325
            shift-left: string[] [] -> [w346]
            shift-right: [w348] -> w324
            shift-left: string[] [] -> [w345]
            tunnel: w318 -> [w358]
            tunnel: w323 -> [w350]
            tunnel: w322 -> [w351]
            tunnel: w321 -> [w352]
            tunnel: w320 -> [w355]
            tunnel: w319 -> [w354]
            tunnel: w308 -> [w368]
            tunnel: w307 -> [w356]
            tunnel: w306 -> [w353]
            i -> [w357]
            # "列定义：0（ID）1（时间/10us）2（0字节）3（1字节）4（2字节）5（3字节）6（4字节）7（5字节）8（6字节）9（7字节）"
            n118 = xnode "匹配正则表达式"("输入字符串"=w369, "正则表达式"=w368) -> ("子匹配 1"=w367:string, "子匹配 2"=w366:string, "子匹配 3"=w365:string, "子匹配 4"=w363:string, "子匹配 5"=w344:string, "子匹配 6"=w332:string)  [unwired: 4 in, 5 out]
            n119 = Decimal String To Number(string=w367) -> (number=w384:i32)  [unwired: 2 in, 1 out]
            n120 = Decimal String To Number(string=w365) -> (number=w364:i32)  [unwired: 2 in, 1 out]
            n121 = Fract/Exp String To Number(string=w363) -> (number=w361:dbl)  [unwired: 3 in, 1 out]
            n122 = Subtract(x=w384, y=w383) -> (x-y=w382:i32)
            n123 = Decimal String To Number(string=w366) -> (number=w380:i32)  [unwired: 2 in, 1 out]
            n124 = Divide(x=w361, y=1000.0) -> (x/y=w360:dbl)
            n125 = Add(x=w364, y=w360) -> (x+y=w359:dbl)
            n126 = Multiply(x=w382, y=3600) -> (x*y=w375:i32)
            n127 = Subtract(x=w380, y=w379) -> (x-y=w378:i32)
            n128 = call "IDandCal.vi"("ID列表In"=w346, "数量统计in"=w345, "ID输入"=w344, "偏移量(0)"=2) -> ("ID列表"=w347:string[], "数量统计"=w348:string[], "ID输出"=w334:u32)  [unwired: 3 in]
            n129 = Subtract(x=w359, y=w374) -> (x-y=w373:dbl)
            n130 = Multiply(x=w378, y=60) -> (x*y=w376:i32)
            n131 = call "TipsWhenDecodeCANdata.vi"("ProgressBar"=w350, "AllRowsNum"=w358, "i"=w357, "ProgressNum"=w351, "Language"=w353, "Tips"=w355, "MessageLinCnt"=w356, "txtAllRowsNum"=w354, "RowsLevel"=w352) -> ()  [unwired: 7 in]
            n132 = Compound Arithmetic op=ADD(w373, w376, w375) -> (w372:dbl)
            n133 = Multiply(x=w372, y=100000.0) -> (x*y=w370:dbl)
            n134 = To Unsigned Long Integer(number=w370) -> (unsigned 32bit integer=w333:u32)
            n135 = call "Datas2Bytes.vi"("DATAs"=w332) -> ("Data5"=w338:u32, "Data4"=w339:u32, "Data3"=w340:u32, "Data2"=w341:u32, "Data6"=w337:u32, "Data1"=w342:u32, "Data7"=w336:u32, "Data0"=w343:u32)  [unwired: 3 in]
            n136 = Build Array(w334, w333, w343, w342, w341, w340, w339, w338, w337, w336) -> (w335:u32[])
          }
        }
        frame False {
          w508 = "\\D*\\s*(\\d+\\.\\d+)\\s+(\\S+)\\s+\\S+\\s+\\S+\\s+\\S+\\s+"
          n137 = Index Array(array=w509, index=0 ("索引")) -> (element=w511:string)
          n138 = xnode "匹配正则表达式"("输入字符串"=w511, "正则表达式"=w508) -> ("子匹配 1"=w507:string)  [unwired: 4 in, 6 out]
          n139 = Fract/Exp String To Number(string=w507) -> (number=w506:dbl)  [unwired: 3 in, 1 out]
          n140 = for {
            tunnel: w509 -> [w673] mode=indexing
            tunnel: w506 -> [w676]
            tunnel: [w649] -> w524 mode=indexing
            shift-right: [w660] -> w521
            shift-left: string[] [] -> [w659]
            shift-right: [w661] -> w520
            shift-left: string[] [] -> [w658]
            tunnel: w514 -> [w671]
            tunnel: w519 -> [w663]
            tunnel: w518 -> [w664]
            tunnel: w517 -> [w665]
            tunnel: w516 -> [w668]
            tunnel: w515 -> [w667]
            tunnel: w508 -> [w672]
            tunnel: w513 -> [w669]
            tunnel: w512 -> [w666]
            i -> [w670]
            # "列定义：0（ID）1（时间/10us）2（0字节）3（1字节）4（2字节）5（3字节）6（4字节）7（5字节）8（6字节）9（7字节）"
            n141 = xnode "匹配正则表达式"("输入字符串"=w673, "正则表达式"=w672) -> ("匹配之后"=w642:string, "子匹配 1"=w645:string, "子匹配 2"=w643:string)  [unwired: 4 in, 4 out]
            n142 = Fract/Exp String To Number(string=w645) -> (number=w644:dbl)  [unwired: 3 in, 1 out]
            n143 = call "IDandCal.vi"("ID列表In"=w659, "数量统计in"=w658, "ID输入"=w643, "偏移量(0)"=2) -> ("ID列表"=w660:string[], "数量统计"=w661:string[], "ID输出"=w648:u32)  [unwired: 3 in]
            n144 = Subtract(x=w644, y=w676) -> (x-y=w646:dbl)
            n145 = call "TipsWhenDecodeCANdata.vi"("ProgressBar"=w663, "AllRowsNum"=w671, "i"=w670, "ProgressNum"=w664, "Language"=w666, "Tips"=w668, "MessageLinCnt"=w669, "txtAllRowsNum"=w667, "RowsLevel"=w665) -> ()  [unwired: 7 in]
            n146 = Multiply(x=w646, y=100000.0) -> (x*y=w674:dbl)
            n147 = To Unsigned Long Integer(number=w674) -> (unsigned 32bit integer=w647:u32)
            n148 = call "Datas2Bytes.vi"("DATAs"=w642) -> ("Data5"=w652:u32, "Data4"=w653:u32, "Data3"=w654:u32, "Data2"=w655:u32, "Data6"=w651:u32, "Data1"=w656:u32, "Data7"=w650:u32, "Data0"=w657:u32)  [unwired: 3 in]
            n149 = Build Array(w648, w647, w657, w656, w655, w654, w653, w652, w651, w650) -> (w649:u32[])
          }
        }
      }
    }
    frame "     index           time           Name             ID        Type      Format  Len      Data" {
      w924 = "\\s*\\d+\\s+(\\d+)\\.(\\d+)\\.(\\d+)\\s+\\S+\\s+(\\S+)\\s+\\S+\\s+\\S+\\s+\\d+\\s+(.*)$"
      # "这是广成ECANTools的txt文件"
      n150 = Index Array(array=w947, index (col)=0 ("禁用的索引 (列)")) -> (element=w944:string[])  [unwired: 1 in]
      n151 = Array Size(array=w944) -> (size(s)=w933:i32)
      n152 = Quotient & Remainder(x=w933, y=100000) -> (floor(x/y)=w936:i32)  [unwired: 1 out]
      n153 = Index Array(array=w944, index=0 ("索引")) -> (element=w929:string)
      n154 = xnode "匹配正则表达式"("输入字符串"=w929, "正则表达式"=w924) -> ("子匹配 1"=w923:string, "子匹配 2"=w921:string, "子匹配 3"=w917:string)  [unwired: 4 in, 5 out]
      n155 = Number To Decimal String(number=w933) -> (decimal integer string=w934:string)  [unwired: 1 in]
      n156 = call "ReadBaseTime.vi"("文件时间？(F)"=TRUE ("文件时间？"), "时间字符"=w914, "日期字符"=w930) -> ("基时间簇"=w927:T1)  [unwired: 6 in]
      n157 = Fract/Exp String To Number(string=w917) -> (number=w932:dbl)  [unwired: 3 in, 1 out]
      n158 = property class="Clust (严格)"(reference=w928, "Value"=w927) -> ()  [unwired: 1 in, 2 out]
      n159 = Divide(x=w932, y=1000000.0) -> (x/y=w916:dbl)
      n160 = Decimal String To Number(string=w923) -> (number=w922:i32)  [unwired: 2 in, 1 out]
      n161 = Decimal String To Number(string=w921) -> (number=w919:i32)  [unwired: 2 in, 1 out]
      n162 = Divide(x=w919, y=1000.0) -> (x/y=w918:dbl)
      n163 = Compound Arithmetic op=ADD(w922, w918, w916) -> (w915:dbl)
      n164 = for {
        tunnel: w944 -> [w1100] mode=indexing
        tunnel: [w1110] -> w948 mode=indexing
        shift-right: [w1105] -> w941
        shift-left: string[] [] -> [w1106]
        shift-right: [w1102] -> w940
        shift-left: string[] [] -> [w1103]
        tunnel: w933 -> [w1098]
        tunnel: w939 -> [w1090]
        tunnel: w938 -> [w1091]
        tunnel: w936 -> [w1092]
        tunnel: w935 -> [w1095]
        tunnel: w934 -> [w1094]
        tunnel: w924 -> [w1099]
        tunnel: w926 -> [w1096]
        tunnel: w925 -> [w1093]
        shift-right: [w1076] -> _
        shift-left: w915 -> [w1077]
        i -> [w1097]
        # "GC的时间是累加"
        # "列定义：0（ID）1（时间/10us）2（0字节）3（1字节）4（2字节）5（3字节）6（4字节）7（5字节）8（6字节）9（7字节）"
        n165 = xnode "匹配正则表达式"("输入字符串"=w1100, "正则表达式"=w1099) -> ("子匹配 1"=w1079:string, "子匹配 2"=w1080:string, "子匹配 3"=w1081:string, "子匹配 4"=w1089:string, "子匹配 5"=w1075:string)  [unwired: 4 in, 5 out]
        n166 = Decimal String To Number(string=w1079) -> (number=w1086:i32)  [unwired: 2 in, 1 out]
        n167 = Fract/Exp String To Number(string=w1081) -> (number=w1088:dbl)  [unwired: 3 in, 1 out]
        n168 = Divide(x=w1088, y=1000000.0) -> (x/y=w1082:dbl)
        n169 = Decimal String To Number(string=w1080) -> (number=w1084:i32)  [unwired: 2 in, 1 out]
        n170 = call "IDandCal.vi"("ID列表In"=w1106, "数量统计in"=w1103, "ID输入"=w1089, "偏移量(0)"=0) -> ("ID列表"=w1105:string[], "数量统计"=w1102:string[], "ID输出"=w1104:u32)  [unwired: 3 in]
        n171 = Divide(x=w1084, y=1000.0) -> (x/y=w1083:dbl)
        n172 = call "TipsWhenDecodeCANdata.vi"("ProgressBar"=w1090, "AllRowsNum"=w1098, "i"=w1097, "ProgressNum"=w1091, "Language"=w1093, "Tips"=w1095, "MessageLinCnt"=w1096, "txtAllRowsNum"=w1094, "RowsLevel"=w1092) -> ()  [unwired: 7 in]
        n173 = Compound Arithmetic op=ADD(w1086, w1083, w1082) -> (w1078:dbl)
        n174 = Add(x=w1077, y=w1078) -> (x+y=w1076:dbl)
        n175 = call "Datas2Bytes.vi"("DATAs"=w1075) -> ("Data5"=w1069:u32, "Data4"=w1070:u32, "Data3"=w1071:u32, "Data2"=w1072:u32, "Data6"=w1068:u32, "Data1"=w1073:u32, "Data7"=w1067:u32, "Data0"=w1074:u32)  [unwired: 3 in]
        n176 = Multiply(x=w1076, y=100000.0) -> (x*y=w1108:dbl)
        n177 = To Unsigned Long Integer(number=w1108) -> (unsigned 32bit integer=w1107:u32)
        n178 = Build Array(w1104, w1107, w1074, w1073, w1072, w1071, w1070, w1069, w1068, w1067) -> (w1110:u32[])
      }
    }
    frame "WRITE_TIME                GROUP_IDDEVICE_TYPE         DEVICE_IDCHANNEL_IDCAN/CANFDCAN_FD_FLAGTX/RX   TX_TYPE RX_TIMESTAMP      SYS_MS            RESERVEDPAD(HEX)      CAN_ID(HEX)FORMAT  FRAME_TYPEDLC     __PAD   __RES0  __RES1  DATA(HEX)" {
      w1238 = 0 ("禁用的索引 (列)")
      n179 = Index Array(array=w1237, index (col)=13 ("禁用的索引 (列)")) -> (element=w1265:string[])  [unwired: 1 in]
      n180 = Index Array(array=w1237, index (col)=10 ("禁用的索引 (列)")) -> (element=w1256:string[])  [unwired: 1 in]
      n181 = Index Array(array=w1237, index (col)=20 ("禁用的索引 (列)")) -> (element=w1261:string[])  [unwired: 1 in]
      n182 = Index Array(array=w1237, index (col)=w1238) -> (element=w1239:string[])  [unwired: 1 in]
      n183 = Array Size(array=w1256) -> (size(s)=w1241:i32)
      n184 = Index Array(array=w1239, index=w1238) -> (element=w1236:string)
      n185 = Index Array(array=w1256, index=0 ("索引")) -> (element=w1235:string)
      n186 = Decimal String To Number(string=w1235, offset=1 ("偏移量")) -> (offset past number=w1253:i32, number=w1257:i32)  [unwired: 1 in]
      n187 = Increment(x=w1253) -> (x+1=w1254:i32)
      n188 = call "ReadBaseTime.vi"("时间字符"=w1235, "日期字符"=w1236) -> ("基时间簇"=w1233:T1)  [unwired: 7 in]
      n189 = Quotient & Remainder(x=w1241, y=100000) -> (floor(x/y)=w1244:i32)  [unwired: 1 out]
      n190 = Decimal String To Number(string=w1235, offset=w1254) -> (offset past number=w1255:i32, number=w1258:i32)  [unwired: 1 in]
      n191 = property class="Clust (严格)"(reference=w1234, "Value"=w1233) -> ()  [unwired: 1 in, 2 out]
      n192 = Increment(x=w1255) -> (x+1=w1259:i32)
      n193 = Number To Decimal String(number=w1241) -> (decimal integer string=w1242:string)  [unwired: 1 in]
      n194 = Fract/Exp String To Number(string=w1235, offset=w1259) -> (number=w1260:dbl)  [unwired: 2 in, 1 out]
      n195 = for {
        tunnel: w1256 -> [w1301] mode=indexing
        tunnel: w1257 -> [w1311]
        tunnel: w1258 -> [w1307]
        tunnel: w1260 -> [w1299]
        tunnel: w1261 -> [w1267] mode=indexing
        tunnel: [w1270] -> w1266 mode=indexing
        shift-right: [w1282] -> w1249
        shift-left: string[] [] -> [w1281]
        shift-right: [w1283] -> w1248
        shift-left: string[] [] -> [w1280]
        tunnel: w1265 -> [w1279] mode=indexing
        tunnel: w1241 -> [w1293]
        tunnel: w1247 -> [w1285]
        tunnel: w1246 -> [w1286]
        tunnel: w1244 -> [w1290]
        tunnel: w1243 -> [w1288]
        tunnel: w1242 -> [w1292]
        tunnel: w1232 -> [w1287]
        tunnel: w1231 -> [w1289]
        i -> [w1291]
        # "列定义：0（ID）1（时间/10us）2（0字节）3（1字节）4（2字节）5（3字节）6（4字节）7（5字节）8（6字节）9（7字节）"
        n196 = Decimal String To Number(string=w1301, offset=1 ("偏移量")) -> (offset past number=w1313:i32, number=w1312:i32)  [unwired: 1 in]
        n197 = Increment(x=w1313) -> (x+1=w1314:i32)
        n198 = Subtract(x=w1312, y=w1311) -> (x-y=w1310:i32)
        n199 = Decimal String To Number(string=w1301, offset=w1314) -> (offset past number=w1315:i32, number=w1308:i32)  [unwired: 1 in]
        n200 = Increment(x=w1315) -> (x+1=w1302:i32)
        n201 = Multiply(x=w1310, y=3600) -> (x*y=w1303:i32)
        n202 = Subtract(x=w1308, y=w1307) -> (x-y=w1306:i32)
        n203 = Fract/Exp String To Number(string=w1301, offset=w1302) -> (number=w1300:dbl)  [unwired: 2 in, 1 out]
        n204 = call "TipsWhenDecodeCANdata.vi"("ProgressBar"=w1285, "AllRowsNum"=w1293, "i"=w1291, "ProgressNum"=w1286, "Language"=w1289, "Tips"=w1288, "MessageLinCnt"=w1287, "txtAllRowsNum"=w1292, "RowsLevel"=w1290) -> ()  [unwired: 7 in]
        n205 = call "IDandCal.vi"("ID列表In"=w1281, "数量统计in"=w1280, "ID输入"=w1279, "偏移量(0)"=2) -> ("ID列表"=w1282:string[], "数量统计"=w1283:string[], "ID输出"=w1268:u32)  [unwired: 3 in]
        n206 = Subtract(x=w1300, y=w1299) -> (x-y=w1298:dbl)
        n207 = Multiply(x=w1306, y=60) -> (x*y=w1304:i32)
        n208 = Compound Arithmetic op=ADD(w1298, w1304, w1303) -> (w1297:dbl)
        n209 = call "Datas2Bytes.vi"("DATAs"=w1267) -> ("Data5"=w1273:u32, "Data4"=w1274:u32, "Data3"=w1275:u32, "Data2"=w1276:u32, "Data6"=w1272:u32, "Data1"=w1277:u32, "Data7"=w1271:u32, "Data0"=w1278:u32)  [unwired: 3 in]
        n210 = Multiply(x=w1297, y=100000.0) -> (x*y=w1295:dbl)
        n211 = To Unsigned Long Integer(number=w1295) -> (unsigned 32bit integer=w1269:u32)
        n212 = Build Array(w1268, w1269, w1278, w1277, w1276, w1275, w1274, w1273, w1272, w1271) -> (w1270:u32[])
      }
    }
  }
  "重构的Data数组" <- w26
  "报文ID" <- w19
  "统计数量" <- w18
  n213 = Build Array(w19, w18) -> (w23:string[][])
  n214 = Transpose 2D Array(2D array=w23) -> (transposed array=w22:string[][])
  n215 = Insert Into Array(array=w22, index (row)=0 ("索引 (行)"), new element=string[] ["CAN报文", "数量"]) -> (→"CAN报文统计":string[][])  [unwired: 1 in]
